vi "DCMotorSim_New_Plant.vi"(8 "MeasurementStdDev":T2=[[0.0], [0.0]], 9 "Gearing":dbl=1.0, 10 "GearBox":T3 {"Jr_KgM2" format="%13.5p"; "L_H" format="%13.5p"; "Kt_NMPerAmp" format="%13.5p"; "KvINV_RadPerSecPerVolt" format="%13.5p"; "R_Ohms" format="%13.5p"; "FreeSpeed_RadPerSec" format="%13.5p"; "FreeCurrent_Amps" format="%13.5p"; "StallCurrent_Amps" format="%13.5p"; "StallTorque_NM" format="%13.5p"; "nominalVoltage_Volts" format="%13.5p"}, 11 "Plant":T1) -> (0 "Error":bool, 3 "DCMotorSim":T4 {"GearBox"."Jr_KgM2" format="%13.5p"; "GearBox"."L_H" format="%13.5p"; "GearBox"."Kt_NMPerAmp" format="%13.5p"; "GearBox"."KvINV_RadPerSecPerVolt" format="%13.5p"; "GearBox"."R_Ohms" format="%13.5p"; "GearBox"."FreeSpeed_RadPerSec" format="%13.5p"; "GearBox"."FreeCurrent_Amps" format="%13.5p"; "GearBox"."StallCurrent_Amps" format="%13.5p"; "GearBox"."StallTorque_NM" format="%13.5p"; "GearBox"."nominalVoltage_Volts" format="%13.5p"})   [LabVIEW 2019, in "Trajectory_Library.lvlib"]
doc: "Creates a simulated DC Motor mechanism.\n \nInputs:\n - plant -- The linear system.\n - gearbox -- The motor definition including the type of and number of motors.\n - gearing -- The gearing of the flywheel (numbers greater than 1 represent reductions).\n - measurementStdDevs -- The standard deviations of the measurements. <2,1> Default: ( 0.0, 0.0 )\n\nOutputs:\n - outDCMotorlSim -- Updated data cluster\n - Error -- If TRUE, an error occured."
uses:
  Trajectory_Library.lvlib
  TypeDef/DCMOTOR_SIM.ctl
  TypeDef/LINEAR_SYSTEM_SIM.ctl
  TypeDef/LINEAR_SYSTEM.ctl
  <vilib>/Analysis/Matrix/Datatypes/RealMatrix.ctl
  TypeDef/DCMOTOR.CTL
  <vilib>/Analysis/Matrix/NI_Matrix.lvlib
panel:
  # "<2 1>"
  # "<States,States>"
  # "<States,Inputs>"
  # "<Outputs,States>"
  # "<Outputs,Inputs>"
  # "<States, 1>"
  # "<Outputs, 1>"
  # "<Inputs, 1>"
  # "<Outputs, 1>"
  # "<States,States>"
  # "<States,Inputs>"
  # "<Outputs,States>"
  # "<Outputs,Inputs>"
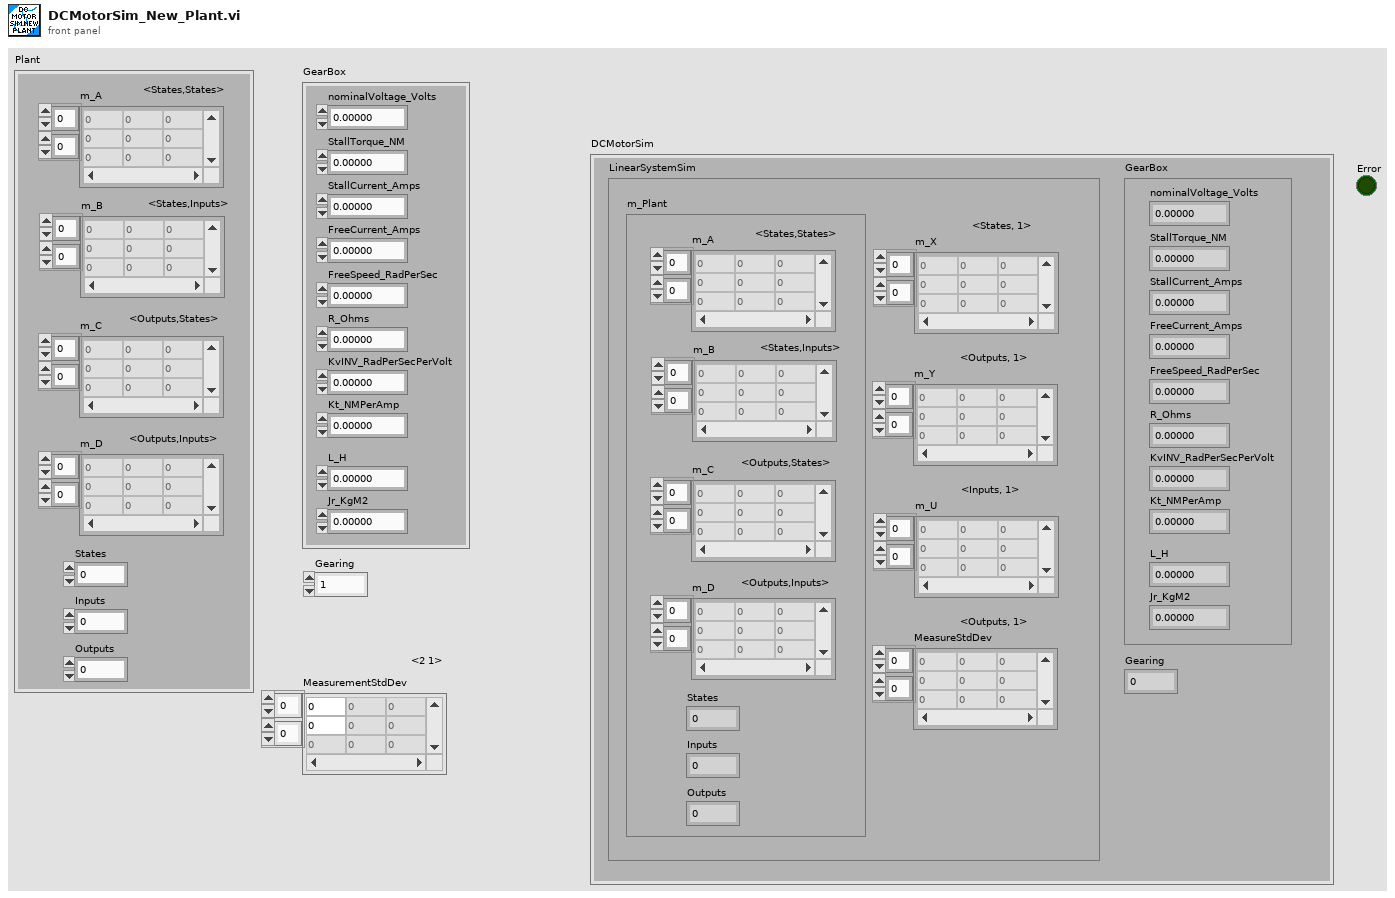
[diagram p1: front panel]
types:
  T1 = typedef "Trajectory_Library.lvlib/LINEAR_SYSTEM.ctl" = cluster{"m_A":T2, "m_B":T2, "m_C":T2, "m_D":T2, "States":i32, "Inputs":i32, "Outputs":i32}
  T2 = typedef "NI_Matrix.lvlib/RealMatrix.ctl" = dbl[][]
  T3 = typedef "Trajectory_Library.lvlib/DCMOTOR.CTL" = cluster{"nominalVoltage_Volts":dbl, "StallTorque_NM":dbl, "StallCurrent_Amps":dbl, "FreeCurrent_Amps":dbl, "FreeSpeed_RadPerSec":dbl, "R_Ohms":dbl, "KvINV_RadPerSecPerVolt":dbl, "Kt_NMPerAmp":dbl, "L_H":dbl, "Jr_KgM2":dbl}
  T4 = typedef "Trajectory_Library.lvlib/DCMOTOR_SIM.ctl" = cluster{"LinearSystemSim":T5, "GearBox":T3, "Gearing":dbl}
  T5 = typedef "Trajectory_Library.lvlib/LINEAR_SYSTEM_SIM.ctl" = cluster{"m_Plant":T1, "m_X":T2, "m_Y":T2, "m_U":T2, "MeasureStdDev":T2}
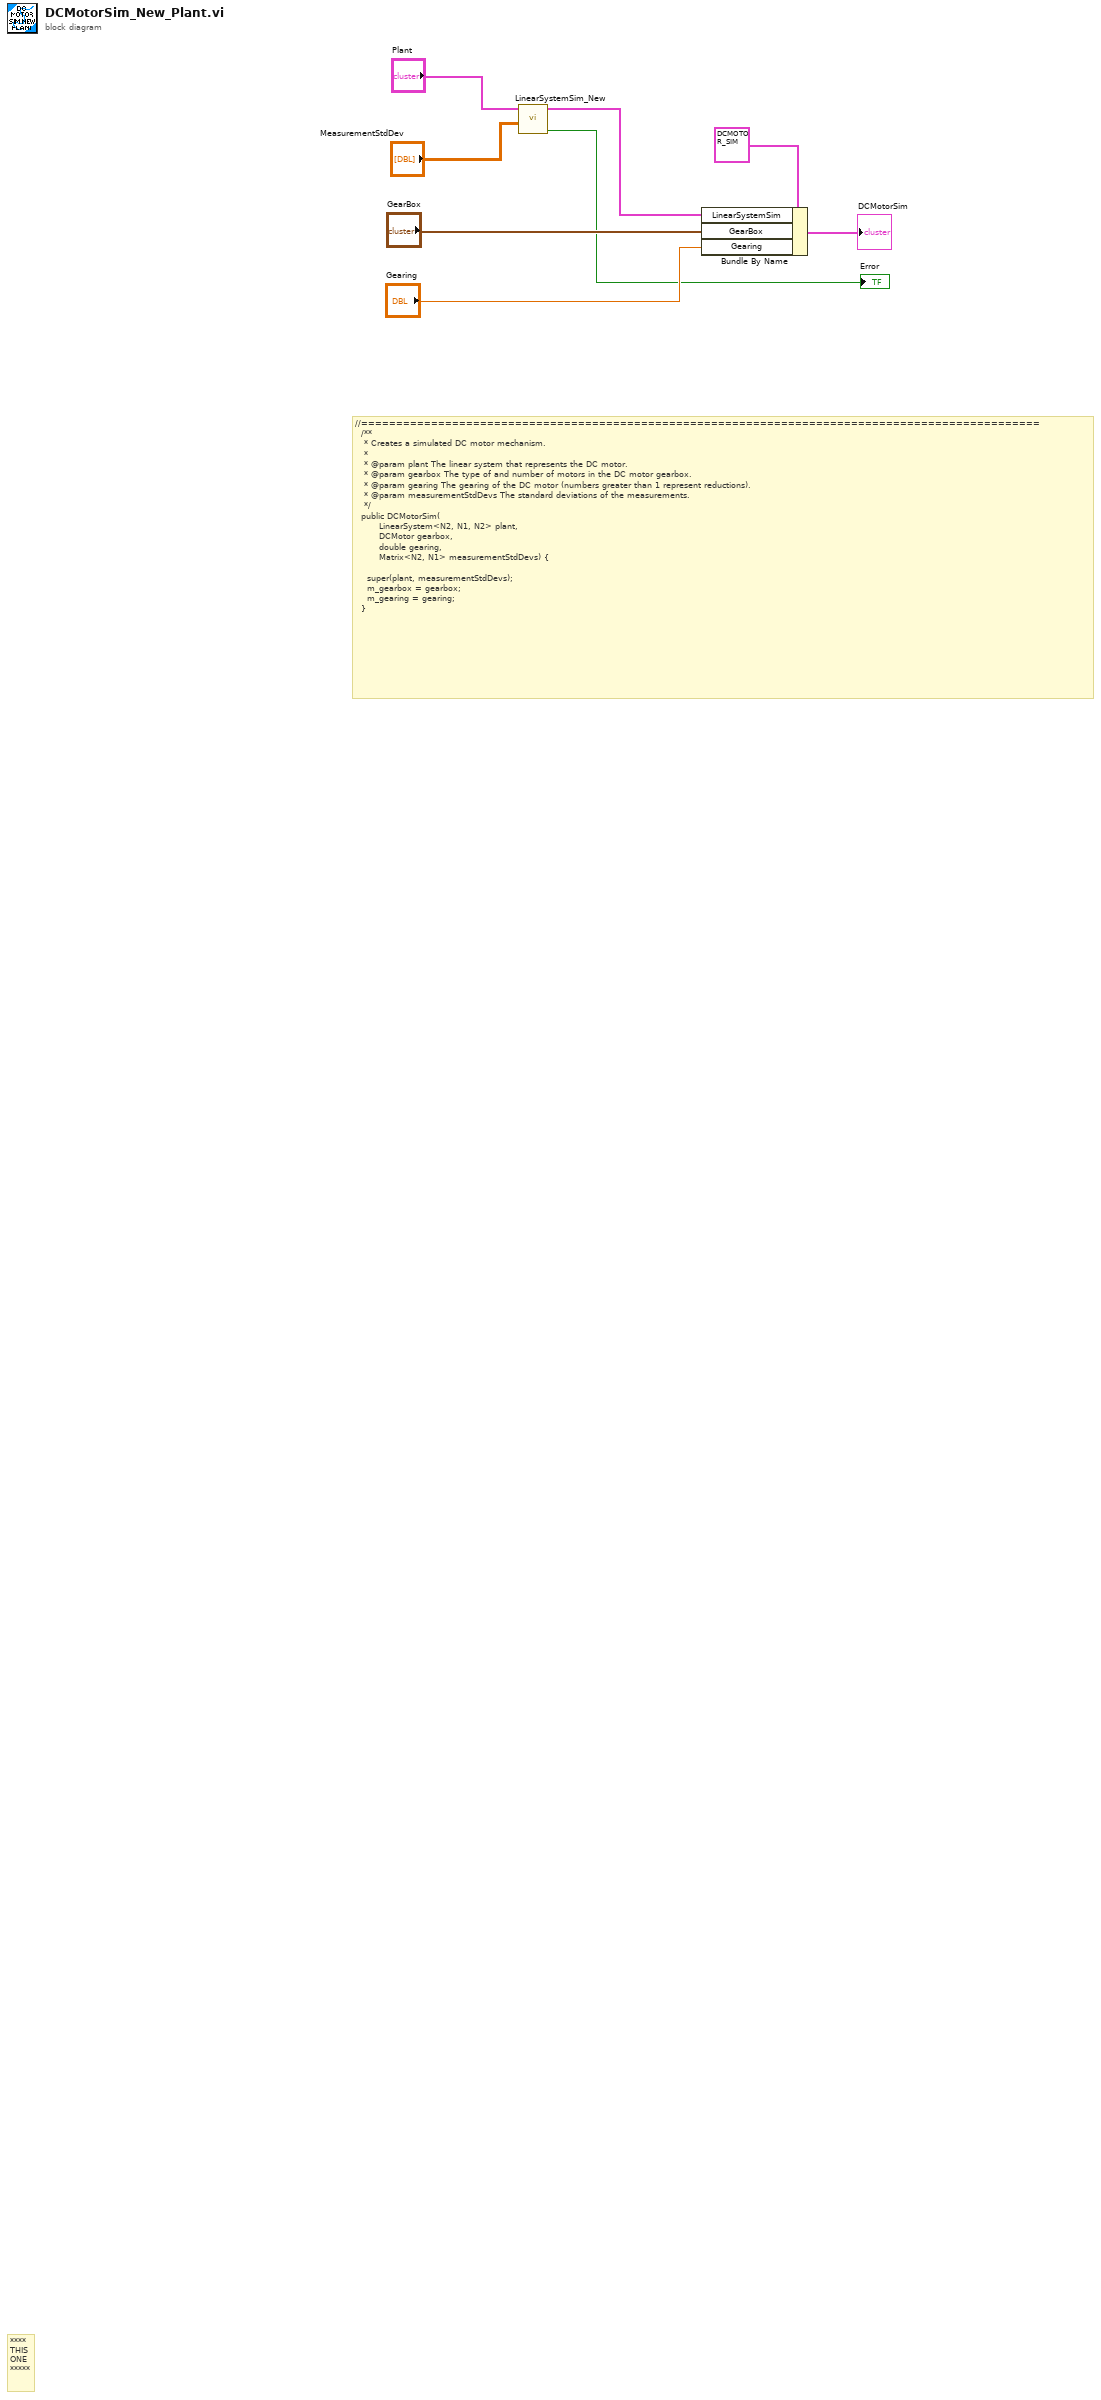
[diagram p0: block diagram]
diagram:
  # "//=================================================================================================\n  /**\n   * Creates a simulated DC motor mechanism.\n   *\n   * @param plant The linear system that represents the DC motor.\n   * @param gearbox The type of and number of motors in the DC motor gearbox.\n   * @param gearing The gearing of the DC motor (numbers greater than 1 represent reductions).\n   * @param measurementStdDevs The standard deviations of the measurements.\n   */\n  public DCMotorSim(\n      \t\tLinearSystem<N2, N1, N2> plant,\n      \t\tDCMotor gearbox,\n      \t\tdouble gearing,\n      \t\tMatrix<N2, N1> measurementStdDevs) {\n\n    super(plant, measurementStdDevs);\n    m_gearbox = gearbox;\n    m_gearing = gearing;\n  }"
  # "****\nTHIS\nONE\n*****"
  n1 = call "LinearSystemSim_New.vi"("MeasurementStdDev"="MeasurementStdDev", "System"="Plant") -> ("Size Coerced"=→"Error":bool, "LinearSystemSim"=w4:T5)  [unwired: 8 in]
  n2 = Bundle By Name(cluster=T4 {"LinearSystemSim"={"m_Plant"={"m_A"=[], "m_B"=[], "m_C"=[], "m_D"=[], "States"=0, "Inputs"=0, "Outputs"=0}, "m_X"=[], "m_Y"=[], "m_U"=[], "MeasureStdDev"=[]}, "GearBox"={"nominalVoltage_Volts"=0.0, "StallTorque_NM"=0.0, "StallCurrent_Amps"=0.0, "FreeCurrent_Amps"=0.0, "FreeSpeed_RadPerSec"=0.0, "R_Ohms"=0.0, "KvINV_RadPerSecPerVolt"=0.0, "Kt_NMPerAmp"=0.0, "L_H"=0.0, "Jr_KgM2"=0.0}, "Gearing"=0.0} ("DCMOTOR_SIM"), "LinearSystemSim"=w4, "GearBox"="GearBox", "Gearing"="Gearing") -> (→"DCMotorSim":T4)
